vi "Write panel mode.vi"(8 "error in (no error)":errorcluster, 10 "Enum":T1, 11 "RocketPlotPanel in":refnum<class "RocketPlotPanel.lvclass">) -> (0 "error out":errorcluster, 3 "RocketPlotPanel out":refnum<class "RocketPlotPanel.lvclass">)   [LabVIEW 2021, in "RocketPlot.lvlib" / "RocketPlotPanel.lvclass"]
uses:
  RocketPlotPanel.lvclass
  RocketPlotPanel.lvclass/RocketPlotPanel.ctl
  TypeDefs/panel mode.ctl
  RocketPlot.lvlib
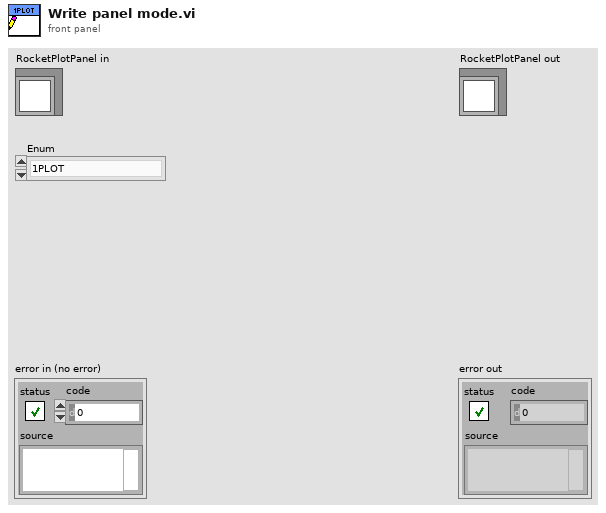
[diagram p1: front panel]
types:
  T1 = typedef "RocketPlot.lvlib/panel mode.ctl" = enum16{"1PLOT", "MPLOT"}
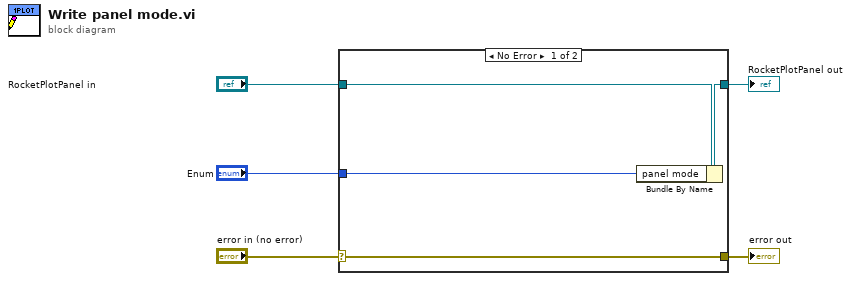
[diagram p0: block diagram]
diagram:
  n1 = case shown="No Error" "error in (no error)" {
    selector: "error in (no error)" -> [w9 w10]
    tunnel: [w9 w10] -> w4
    tunnel: [w7 w11] -> w2
    tunnel: "RocketPlotPanel in" -> [w8 w11]
    tunnel: "Enum" -> [w6 _]
    frame No Error {
      n2 = Bundle By Name(cluster=w8, "panel mode"=w6) -> (w7:refnum<class "RocketPlotPanel.lvclass">)
    }
    frame Error {
    }
  }
  "error out" <- w4
  "RocketPlotPanel out" <- w2
